vi "data sorting unknown simple.vi"(8 "error in":errorcluster, 11 "cycle results cluster IN":T1) -> (0 "error out":errorcluster, 3 "cycle results cluster out":T1)   [LabVIEW 2016]
doc: "Takes a sample type and sorts by sequence"
uses:
  controls/cycle results control.ctl
  <vilib>/Analysis/baseanly.llb/Mean (DBL).vi
  <vilib>/Analysis/NI_AALBase.lvlib
panel:
  out "Array":dbl[][](array[numeric])
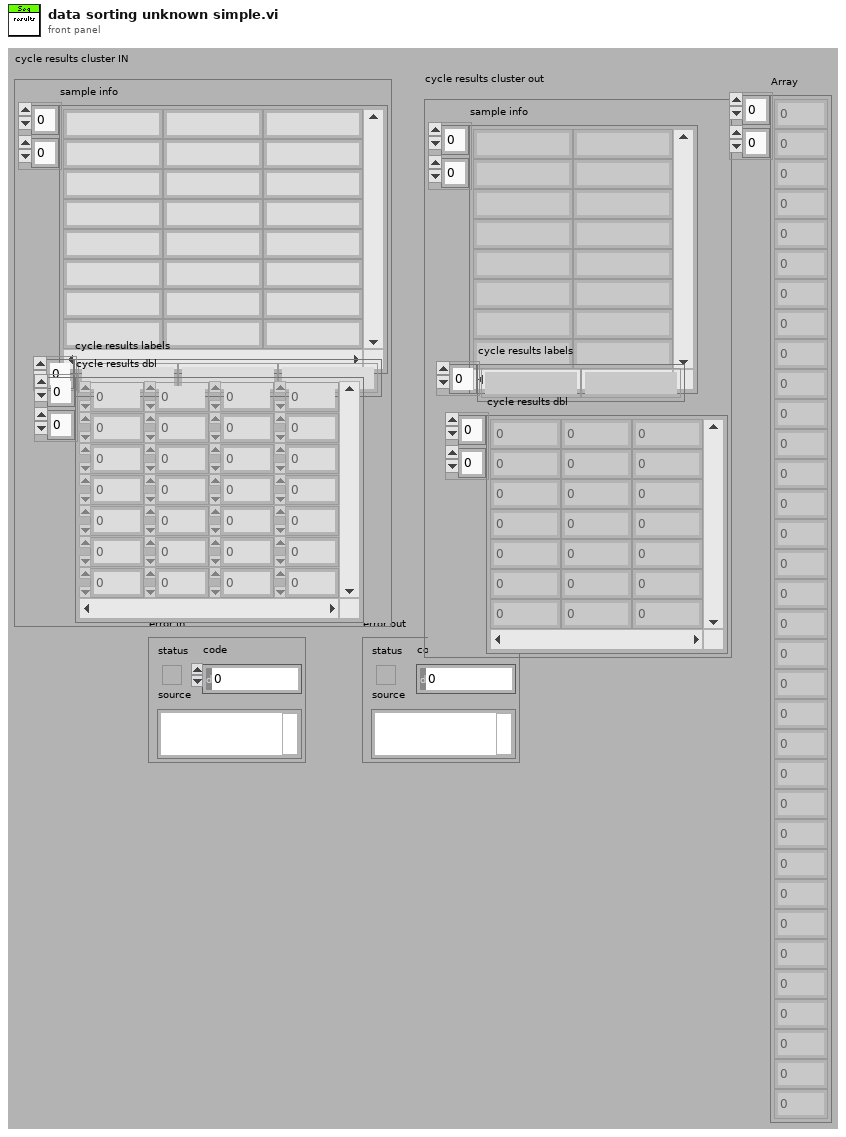
[diagram p1: front panel]
types:
  T1 = typedef "cycle results control.ctl" = cluster{"sample info":string[][], "cycle results labels":string[], "cycle results dbl":dbl[][]}
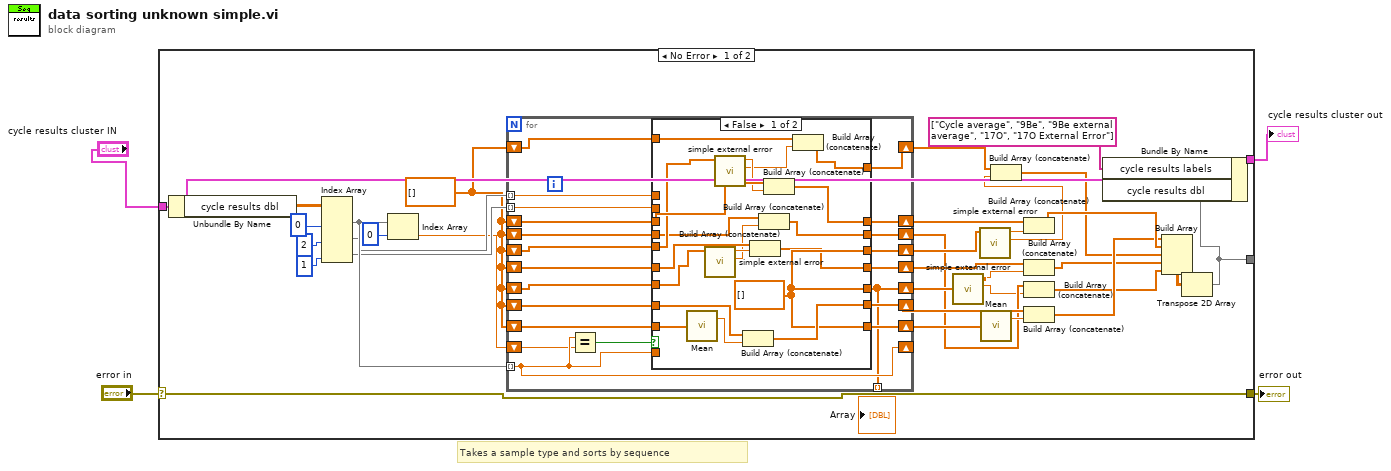
[diagram p0: block diagram]
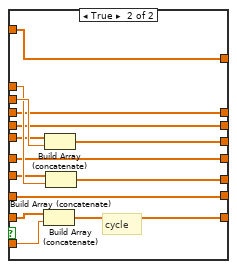
[diagram p2: hidden frame]
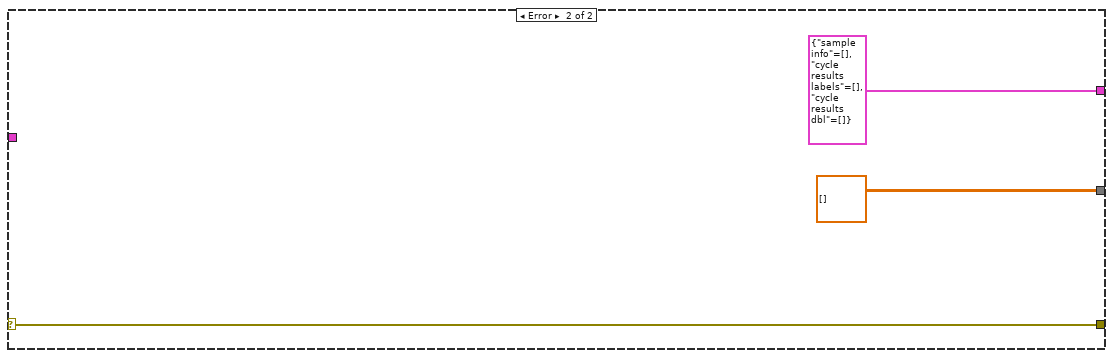
[diagram p3: hidden frame]
diagram:
  # "Takes a sample type and sorts by sequence"
  n1 = case shown="No Error" "error in" {
    selector: "error in" -> [w24 w95]
    tunnel: "cycle results cluster IN" -> [w23 _]
    tunnel: [w19 dbl[][] []] -> _
    tunnel: [w21 T1 {"sample info"=[], "cycle results labels"=[], "cycle results dbl"=[]} ("cycle results cluster IN")] -> w2
    tunnel: [w24 w95] -> w3
    frame No Error {
      w7 = dbl[] []
      n2 = Unbundle By Name(w23) -> ("cycle results dbl"=w33:dbl[][])
      n3 = Index Array(array=w33, index (col) #1=0 ("disabled index (col)"), index (col) #2=2 ("index (col)"), index (col) #3=1 ("index (col)")) -> (element #1=w29:dbl[], element #2=w28:dbl[], element #3=w27:dbl[])  [unwired: 3 in]
      n4 = Index Array(array=w29, index=0) -> (element=w5:dbl)
      n5 = for {
        tunnel: w29 -> [w55] mode=indexing
        shift-right: [w59] -> w35
        shift-left: w7 -> [w58]
        shift-right: [w57] -> w39
        shift-left: w7 -> [w56]
        shift-right: [w55] -> _
        shift-left: w5 -> [w40]
        tunnel: w27 -> [w54] mode=indexing
        tunnel: w28 -> [w53] mode=indexing
        shift-right: [w41] -> w14
        shift-left: w7 -> [w50]
        shift-right: [w52] -> w18
        shift-left: w7 -> [w51]
        shift-right: [w49] -> w36
        shift-left: w7 -> [w47]
        shift-right: [w48] -> w37
        shift-left: w7 -> [w46]
        shift-right: [w45] -> w15
        shift-left: w7 -> [w44]
        shift-right: [w43] -> w12
        shift-left: w7 -> [w42]
        tunnel: [w41] -> w6 mode=indexing
        n6 = Equal?(x=w55, y=w40) -> (x = y?=w60:bool)
        n7 = case shown="False" w60 {
          tunnel: w55 -> [_ w90]
          tunnel: [w75 w93] -> w59
          tunnel: w58 -> [w79 w91]
          tunnel: [w78 w92] -> w57
          tunnel: w56 -> [w77 w92]
          tunnel: w54 -> [_ w89]
          tunnel: w53 -> [_ w88]
          tunnel: [w75 w80] -> w41
          tunnel: [w75 w87] -> w52
          tunnel: w51 -> [w67 w86]
          tunnel: w50 -> [w65 w85]
          tunnel: [w74 w84] -> w49
          tunnel: [w73 w83] -> w48
          tunnel: w47 -> [w72 w84]
          tunnel: w46 -> [w71 w83]
          tunnel: [w70 w82] -> w45
          tunnel: w44 -> [w69 w82]
          tunnel: [w62 w81] -> w43
          tunnel: w42 -> [w61 w81]
          frame False {
            w75 = dbl[] []
            n8 = call-poly <vilib>:"Mean.vi"("X"=w79) -> ("mean"=w76:dbl)  [unwired: 1 out]
            n9 = call "simple external error.vi"("cycle results"=w65) -> ("External error"=w63:dbl, "Sequence result"=w64:dbl)  [unwired: 7 in, 2 out]
            n10 = call "simple external error.vi"("cycle results"=w67) -> ("External error"=w66:dbl, "Sequence result"=w68:dbl)  [unwired: 7 in, 2 out]
            n11 = Build Array (concatenate)(w77, w76) -> (w78:dbl[])
            n12 = Build Array (concatenate)(w71, w64) -> (w73:dbl[])
            n13 = Build Array (concatenate)(w61, w63) -> (w62:dbl[])
            n14 = Build Array (concatenate)(w72, w68) -> (w74:dbl[])
            n15 = Build Array (concatenate)(w69, w66) -> (w70:dbl[])
          }
          frame True {
            # "cycle"
            n16 = Build Array (concatenate)(w91, w90) -> (w93:dbl[])
            n17 = Build Array (concatenate)(w86, w89) -> (w87:dbl[])
            n18 = Build Array (concatenate)(w85, w88) -> (w80:dbl[])
          }
        }
      }
      "Array" <- w6
      n19 = call "simple external error.vi"("cycle results"=w14) -> ("External error"=w11:dbl, "Sequence result"=w13:dbl)  [unwired: 7 in, 2 out]
      n20 = call "simple external error.vi"("cycle results"=w18) -> ("External error"=w16:dbl, "Sequence result"=w17:dbl)  [unwired: 7 in, 2 out]
      n21 = call-poly <vilib>:"Mean.vi"("X"=w35) -> ("mean"=w38:dbl)  [unwired: 1 out]
      n22 = Build Array (concatenate)(w15, w16) -> (w10:dbl[])
      n23 = Build Array (concatenate)(w36, w17) -> (w26:dbl[])
      n24 = Build Array (concatenate)(w37, w13) -> (w9:dbl[])
      n25 = Build Array (concatenate)(w12, w11) -> (w8:dbl[])
      n26 = Build Array (concatenate)(w39, w38) -> (w25:dbl[])
      n27 = Build Array(w25, w26, w10, w9, w8) -> (w20:dbl[][])
      n28 = Transpose 2D Array(2D array=w20) -> (transposed array=w19:dbl[][])
      n29 = Bundle By Name(cluster=w23, "cycle results labels"=string[] ["Cycle average", "9Be", "9Be external average", "17O", "17O External Error"], "cycle results dbl"=w19) -> (w21:T1)
    }
    frame Error {
    }
  }
  "error out" <- w3
  "cycle results cluster out" <- w2
